vi "Set Channels.vi"(8 "error in":errorcluster, 10 "Channels":T1[](array[typedef]) format="%.0x", 11 "Execution Unit":T2 {"ReadWrite Channels" format="%.0x"; "Outgoing Channels" format="%.0x"; "Incoming Channels" format="%.0x"}) -> (0 "error out":errorcluster, 3 "Execution Unit out":T2 {"ReadWrite Channels" format="%.0x"; "Outgoing Channels" format="%.0x"; "Incoming Channels" format="%.0x"})   [LabVIEW 2020, in "AIM MIL-STD-1553 Engine.lvlib" / "Interfaces.lvlib"]
uses:
  Interfaces.lvlib
  <vilib>/NI VeriStand/Custom Device API/Custom Device API.lvlib
  Execution Unit/Execution Unit.lvclass
  <vilib>/NI VeriStand/Custom Device API/Custom Device Item Ref.ctl
  Controls/Execution Unit Information.ctl
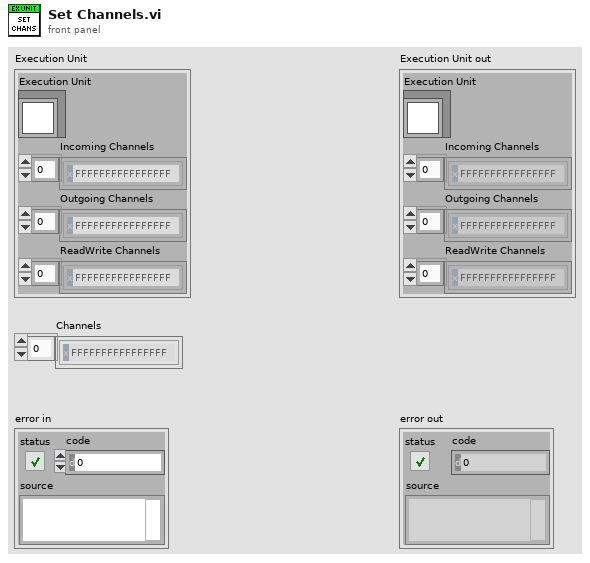
[diagram p1: front panel]
types:
  T1 = typedef "Custom Device API.lvlib/Custom Device Item Ref.ctl" = u64
  T2 = typedef "AIM MIL-STD-1553 Engine.lvlib/Interfaces.lvlib/Execution Unit Information.ctl" = cluster{"Execution Unit":refnum<class "Execution Unit.lvclass">, "Incoming Channels":T1[], "Outgoing Channels":T1[], "ReadWrite Channels":T1[]}
  T3 = typedef "Custom Device API.lvlib/Custom Device Channel.ctl" = cluster{"Type":T4, "Units":string, "Default Value":dbl, "Faultable":bool, "Scalable":bool}
  T4 = typedef "Custom Device API.lvlib/Custom Device Channel Type.ctl" = enum16{"Input", "Output"}
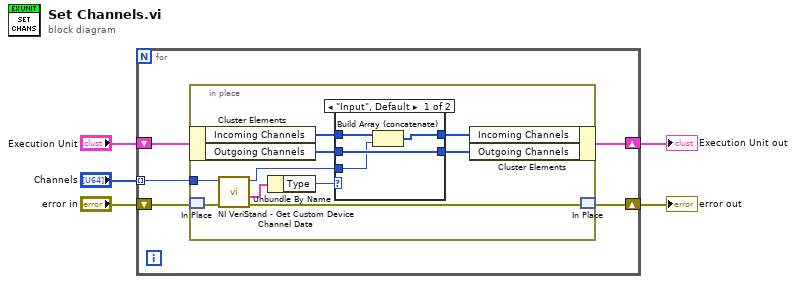
[diagram p0: block diagram]
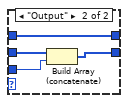
[diagram p2: hidden frame]
diagram:
  n1 = for {
    tunnel: "Channels" -> [w9] mode=indexing
    shift-right: [w6] -> w1
    shift-left: "Execution Unit" -> [w10]
    shift-right: [w7] -> w2
    shift-left: "error in" -> [w8]
    n2 = in-place {
      in-place-border: w9 -> [w20]
      n3 = in-place-cluster #1(w10) -> ("Incoming Channels"=w18:T1[], "Outgoing Channels"=w17:T1[])
      n4 = in-place-match #2(w8) -> (w16:errorcluster)
      n5 = call <vilib>:"NI VeriStand - Get Custom Device Channel Data.vi"("error in (no error)"=w16, "Channel Ref in"=w20) -> ("error out"=w11:errorcluster, "Channel"=w19:T3, "Channel Ref out"=w14:T1)  [unwired: 4 in, 3 out]
      n6 = Unbundle By Name(w19) -> ("Type"=w15:T4)
      n7 = case shown="\"Input\", Default" w15 {
        tunnel: w18 -> [w24 w27]
        tunnel: w17 -> [w23 w28]
        tunnel: w14 -> [w22 w26]
        tunnel: [w21 w27] -> w13
        tunnel: [w23 w25] -> w12
        frame "Input", Default {
          n8 = Build Array (concatenate)(w24, w22) -> (w21:T1[])
        }
        frame "Output" {
          n9 = Build Array (concatenate)(w28, w26) -> (w25:T1[])
        }
      }
      n10 = in-place-cluster #1("Incoming Channels"=w13, "Outgoing Channels"=w12) -> (w6:T2)
      n11 = in-place-match #2(w11) -> (w7:errorcluster)
    }
  }
  "Execution Unit out" <- w1
  "error out" <- w2
